vi "SetUpGage.vi"(0 "Digitizer Settings":T1={"Digitizer delay (us) "=0.0, "rf points per line"=2048, "lines per plane"=128, "Samp Rate (Hz)"=100000000.0, "Additional dig delay (us)"=0.0, "Voltage Scale"=0.4, "Pre-Looks"=0, "Offset delay (us)"=0.0, "bits A/D"=8, "Avg Num"=1, "DigTimeOut"=5.0, "Rel Dig Delay"=0.0, "Dig Ch"=0, "LeCroyCluster"={"LeCroy Channels"=[TRUE, FALSE, FALSE, FALSE], "LC read pt offset"=0.0, "Sweep Avg"=FALSE}, "Main Digitizer"=enum."NI Digitizer", "Dig Config"=enum."Single channel", "Digitizer ID Cluster"={"Acqiris/Alazar/SP ID"=[], "NI Instr Handles"=[], "LeCroy VISA"="", "GaGe Handle"={"Handle"=0, "Sample size"=0, "Resolution"=0, "Offset"=0, "Channels"=0, "Boards"=0}, "ATS Ref"="ATS9350", "Acqiris Address"=["PCI::INSTR0"], "ADQRef"=refnum, "adq_cu_ptr"=refnum}, "Trigger Settings"={"Trig Source"=1, "Trig Coupling"=0, "Trig Slope"=0, "Level (mV)"=1500.0}, "Bulk Acq"=FALSE, "Bulk Start Indexes"=[], "Data Ref RF"=refnum, "NI ID/Channel"=[], "Total Dig CH"=5, "Xtra Ann Trig delay (us)"=10.0, "Fix Z Delay?"=FALSE, "One Way Transmission?"=FALSE, "Data Ref Log"=refnum} {"Trigger Settings"."Trig Slope" items=["Positive", "Negative"]; "Trigger Settings"."Level (mV)" format="%.2f"; "Trigger Settings"."Trig Coupling" items=["DC 1 MOhm", "AC 1 MOhm", "DC 50 Ohm", "AC 50 Ohm"]; "Trigger Settings"."Trig Source" items=["Chan 1", "External"]; "Rel Dig Delay" format="%.2f"; "DigTimeOut" format="%.2f"; "Avg Num" min=1; "Offset delay (us)" format="%.2f"; "Additional dig delay (us)" format="%.2f"; "Digitizer delay (us)" format="%.2f"}, 1 "Vecchio Hitachi?":bool, 3 "Acquisition In":T5, 4 "Attenuation":u8(slide) max=63 scale=0.0..63.0, 5 "Vector Trigger Line":i16=150 min=2 max=315, 6 "Machine Type":enum16{"Hitachi", "B&K 3535", "B&K Hawk"}(ring)) -> (12 "Total Delay (ms)":dbl format="%.2f", 13 "Additional dig delay (ms) out":dbl format="%.2f", 14 "Digitizer Settings Out":T1={"Digitizer delay (us) "=0.0, "rf points per line"=2048, "lines per plane"=128, "Samp Rate (Hz)"=100000000.0, "Additional dig delay (us)"=0.0, "Voltage Scale"=0.4, "Pre-Looks"=0, "Offset delay (us)"=0.0, "bits A/D"=8, "Avg Num"=1, "DigTimeOut"=5.0, "Rel Dig Delay"=0.0, "Dig Ch"=0, "LeCroyCluster"={"LeCroy Channels"=[TRUE, FALSE, FALSE, FALSE], "LC read pt offset"=0.0, "Sweep Avg"=FALSE}, "Main Digitizer"=enum."NI Digitizer", "Dig Config"=enum."Single channel", "Digitizer ID Cluster"={"Acqiris/Alazar/SP ID"=[], "NI Instr Handles"=[], "LeCroy VISA"="", "GaGe Handle"={"Handle"=0, "Sample size"=0, "Resolution"=0, "Offset"=0, "Channels"=0, "Boards"=0}, "ATS Ref"="ATS9350", "Acqiris Address"=["PCI::INSTR0"], "ADQRef"=refnum, "adq_cu_ptr"=refnum}, "Trigger Settings"={"Trig Source"=1, "Trig Coupling"=0, "Trig Slope"=0, "Level (mV)"=1500.0}, "Bulk Acq"=FALSE, "Bulk Start Indexes"=[], "Data Ref RF"=refnum, "NI ID/Channel"=[], "Total Dig CH"=5, "Xtra Ann Trig delay (us)"=10.0, "Fix Z Delay?"=FALSE, "One Way Transmission?"=FALSE, "Data Ref Log"=refnum} {"Trigger Settings"."Trig Slope" items=["Positive", "Negative"]; "Trigger Settings"."Level (mV)" format="%.2f"; "Trigger Settings"."Trig Coupling" items=["DC 1 MOhm", "AC 1 MOhm", "DC 50 Ohm", "AC 50 Ohm"]; "Trigger Settings"."Trig Source" items=["Chan 1", "External"]; "Rel Dig Delay" format="%.2f"; "DigTimeOut" format="%.2f"; "Avg Num" min=1; "Offset delay (us)" format="%.2f"; "Additional dig delay (us)" format="%.2f"; "Digitizer delay (us)" format="%.2f"}, 15 "Attenuation out":u8, 16 "Acquisition Settings Out":T5, 18 "Equivalent round trip\ndelay distance (mm)":dbl format="%.2f", 19 "Voltage Scale (pp) OUT":i16(ring)=5)   [LabVIEW 2022 SP3]
uses:
  <vilib>/Analysis/NI_AALPro.lvlib
  <instrlib>/vi.lib/Platform/portaccess.llb/Out Port8.vi
  <vilib>/Analysis/NI_AALBase.lvlib
  <vilib>/Analysis/baseanly.llb/Mean (DBL).vi
  ProstateDataAcq/-ProstateScanSystem/RFSamplingCluster.ctl
  -DigitizerRoutines/DigitizerID.ctl
  -DigitizerRoutines/DigitizerSettings.ctl
  -DigitizerRoutines/Digitizer.ctl
  -DigitizerRoutines/DigConfig.ctl
  C:/Windows/System32/ADQAPI_dotNet_helper.dll
panel:
  in  "Trigger Settings":T6={"Source"=1, "Coupling"=0, "Slope"=0, "Level (mV)"=1500.0} {"Slope" items=["Positive", "Negative"]; "Level (mV)" format="%.2f"; "Coupling" items=["DC 1 MOhm", "AC 1 MOhm", "DC 50 Ohm", "AC 50 Ohm"]; "Source" items=["Chan 1", "External"]}
  in  "Offset (mV)":dbl
  in  "Channel":u16(ring) items=["Ch 0", "Ch 1"]
  in  "Voltage Scale (pp)":i16(ring)=5
  in  "go to scan type":bool
  in  "ExitSendCmd":bool
  in  "Coupling":u16(ring)=3 items=["DC 1 MOhm", "AC 1 MOhm", "DC 50 Ohm", "AC 50 OHM"]
  in  "Time scale per Div":i32(ring)=7 items=["100 ns", "200 ns", "500 ns", "1 micros", "2 micros", "5 micros", "10 micros", "20 micros", "50 micros", "100 micros", "200 micros"]
  out "Waveform\nGraph":cluster{i32, dbl, dbl[]}(graph)
  out "Error Message":string
  in  "RF data Sampling":T7={"Sampling Rate"=50, "Ref Delay (ms)"=0.0, "rf points per line"=2500} {"Ref Delay (ms)" format="%.2f"}
  # "Digitizer Settings"
  # "Scale Settings"
  # "Need to autoscale if viewing spectrum. Yellow curser used for additional delay.\nRF data is captured between yellow and red lines."
  # "© 2000-2014 Riverside Research Institute"
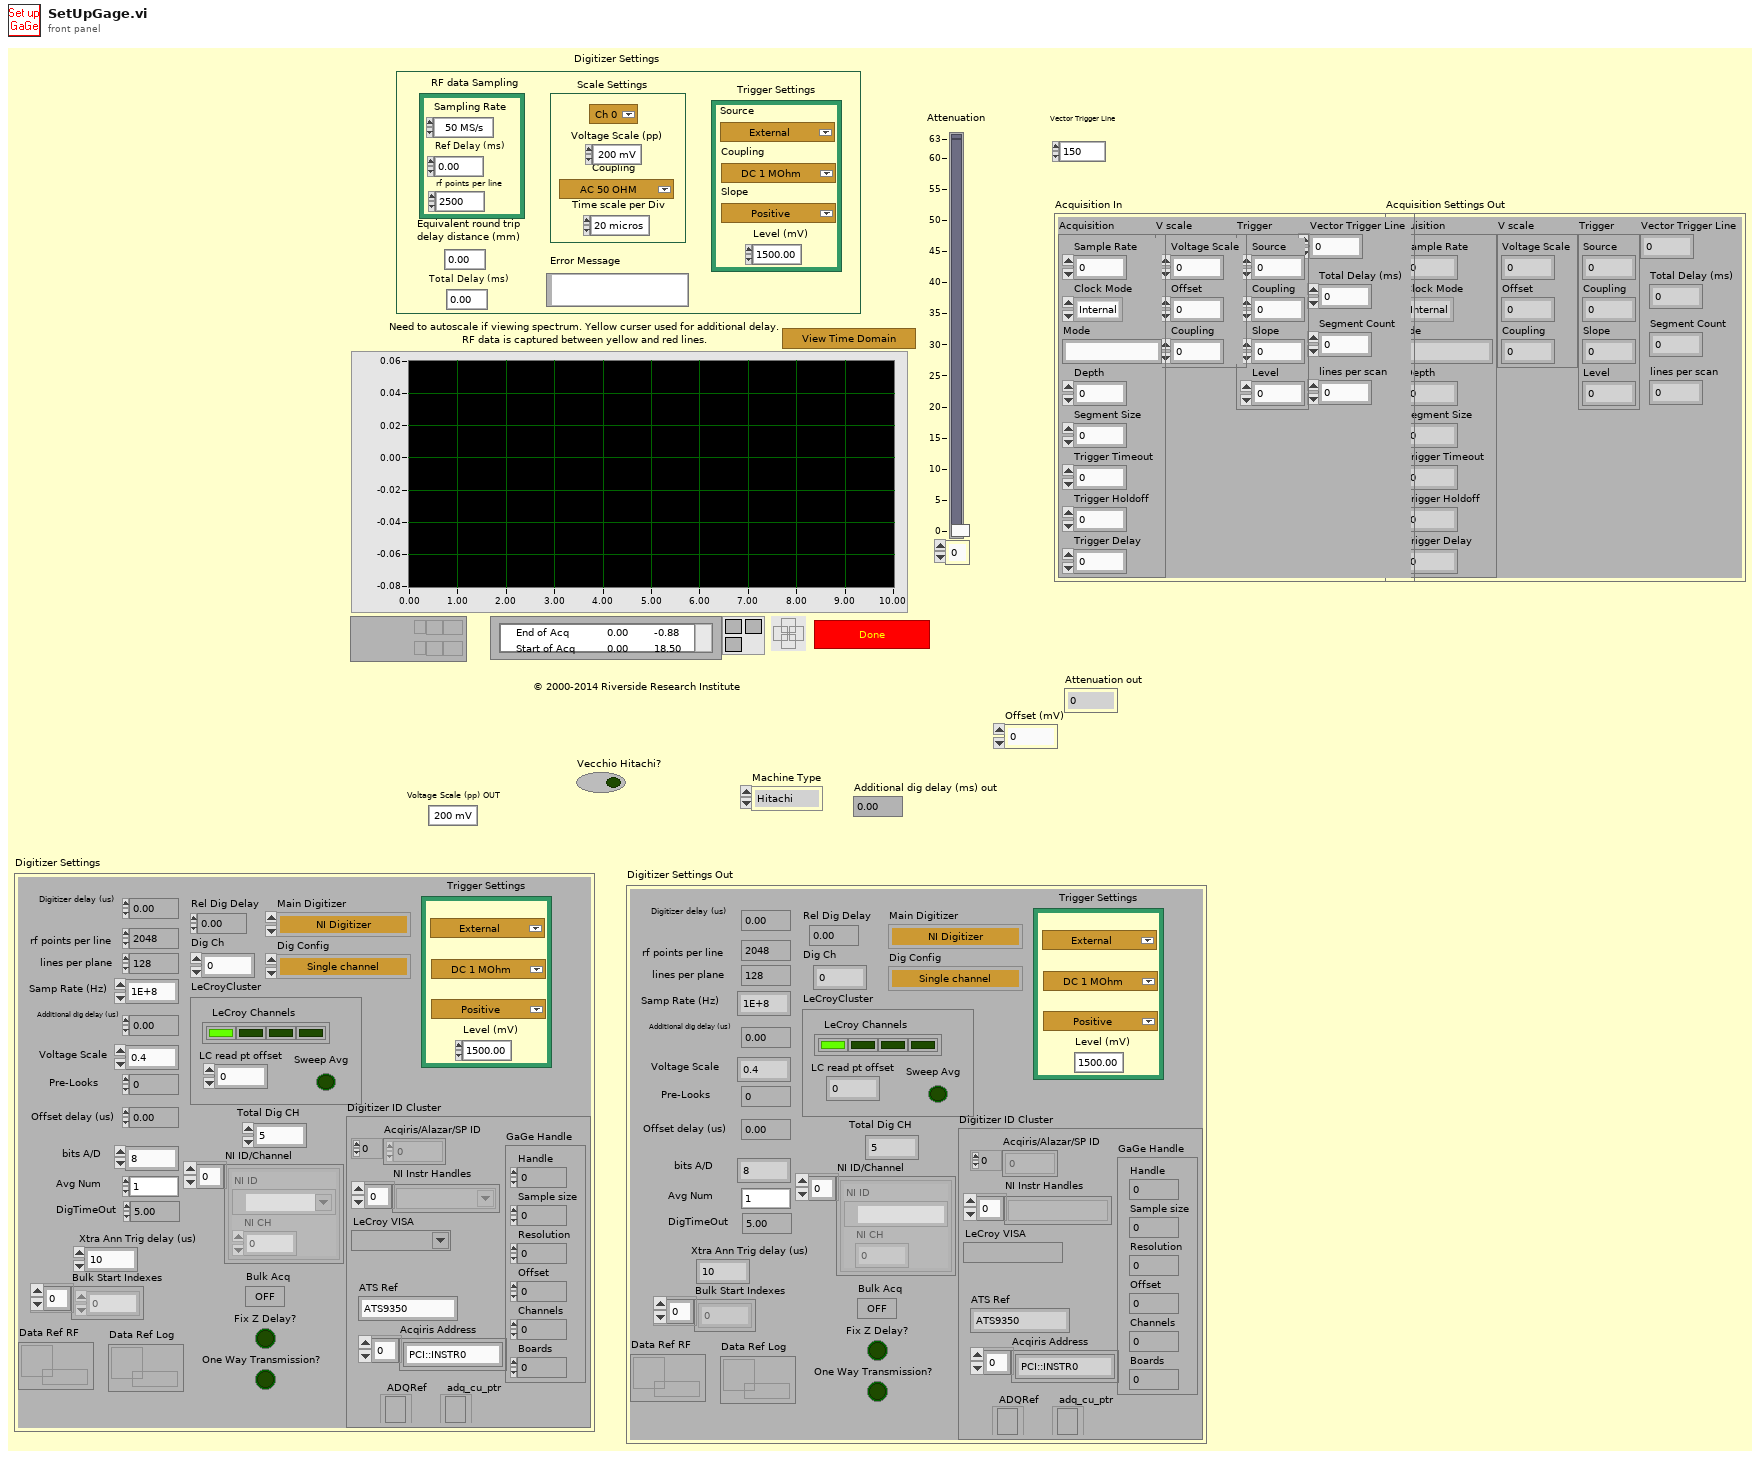
[diagram p1: front panel]
types:
  T1 = typedef "DigitizerSettings.ctl" = cluster{"Digitizer delay (us) ":dbl, "rf points per line":i32, "lines per plane":i32, "Samp Rate (Hz)":dbl, "Additional dig delay (us)":dbl, "Voltage Scale":dbl, "Pre-Looks":i32, "Offset delay (us)":dbl, "bits A/D":i8, "Avg Num":i32, "DigTimeOut":sgl, "Rel Dig Delay":sgl, "Dig Ch":i32, "LeCroyCluster":cluster{"LeCroy Channels":bool[], "LC read pt offset":dbl, "Sweep Avg":bool}, "Main Digitizer":T2, "Dig Config":T3, "Digitizer ID Cluster":T4, "Trigger Settings":cluster{"Trig Source":u16, "Trig Coupling":u16, "Trig Slope":u16, "Level (mV)":dbl}, "Bulk Acq":bool, "Bulk Start Indexes":i32[], "Data Ref RF":refnum<data-value>, "NI ID/Channel":cluster{"NI ID":refnum<k15>, "NI CH":i32}[], "Total Dig CH":i32, "Xtra Ann Trig delay (us)":dbl, "Fix Z Delay?":bool, "One Way Transmission?":bool, "Data Ref Log":refnum<data-value>}
  T2 = typedef "Digitizer.ctl" = enum16{"Acqiris Digitizer", "NI Digitizer", "LeCroy", "GaGe", "AlazarTech", "No Digitizer", "Teledyne"}
  T3 = typedef "DigConfig.ctl" = enum16{"Single channel", "2 Chans w/ 2 Acqiris", "2 Chans w/ 1 Acqiris", "5-CH Pulser New", "5-CH pulser w/ ann array", "5-pass style ann array", "Empty"}
  T4 = typedef "DigitizerID.ctl" = cluster{"Acqiris/Alazar/SP ID":u32[], "NI Instr Handles":refnum<k15>[], "LeCroy VISA":refnum<visa-resource-name>, "GaGe Handle":cluster{"Handle":u32, "Sample size":u32, "Resolution":i32, "Offset":i32, "Channels":u32, "Boards":u32}, "ATS Ref":string, "Acqiris Address":string[], "ADQRef":refnum<k24>, "adq_cu_ptr":refnum<k24>}
  T5 = cluster{"Acquisition":cluster{"Sample Rate":dbl, "Clock Mode":enum16{"Internal", "External", "Reference"}, "Mode":string, "Depth":dbl, "Segment Size":dbl, "Trigger Timeout":dbl, "Trigger Holdoff":dbl, "Trigger Delay":dbl}, "V scale":cluster{"Voltage Scale":i16, "Offset":dbl, "Coupling":u16}, "Trigger":cluster{"Source":u16, "Coupling":u16, "Slope":u16, "Level":dbl}, "Vector Trigger Line":i16, "Total Delay (ms)":dbl, "Segment Count":u32, "lines per scan":i32}
  T6 = cluster{"Source":u16, "Coupling":u16, "Slope":u16, "Level (mV)":dbl}
  T7 = typedef "RFSamplingCluster.ctl" = cluster{"Sampling Rate":u16, "Ref Delay (ms)":dbl, "rf points per line":u16}
  T8 = cluster{"Handle":u32, "Sample size":u32, "Resolution":i32, "Offset":i32, "Channels":u32, "Boards":u32}
  T9 = cluster{"Voltage Scale (pp)":i16, dbl, "Coupling":u16}
  T10 = cluster{"Sample Rate":dbl, "Clock Mode":enum16{"Internal", "External", "Reference"}, "Mode":string, "Depth":dbl, "Segment Size":dbl, "Trigger Timeout":dbl, "Trigger Holdoff":dbl, "Trigger Delay":dbl}
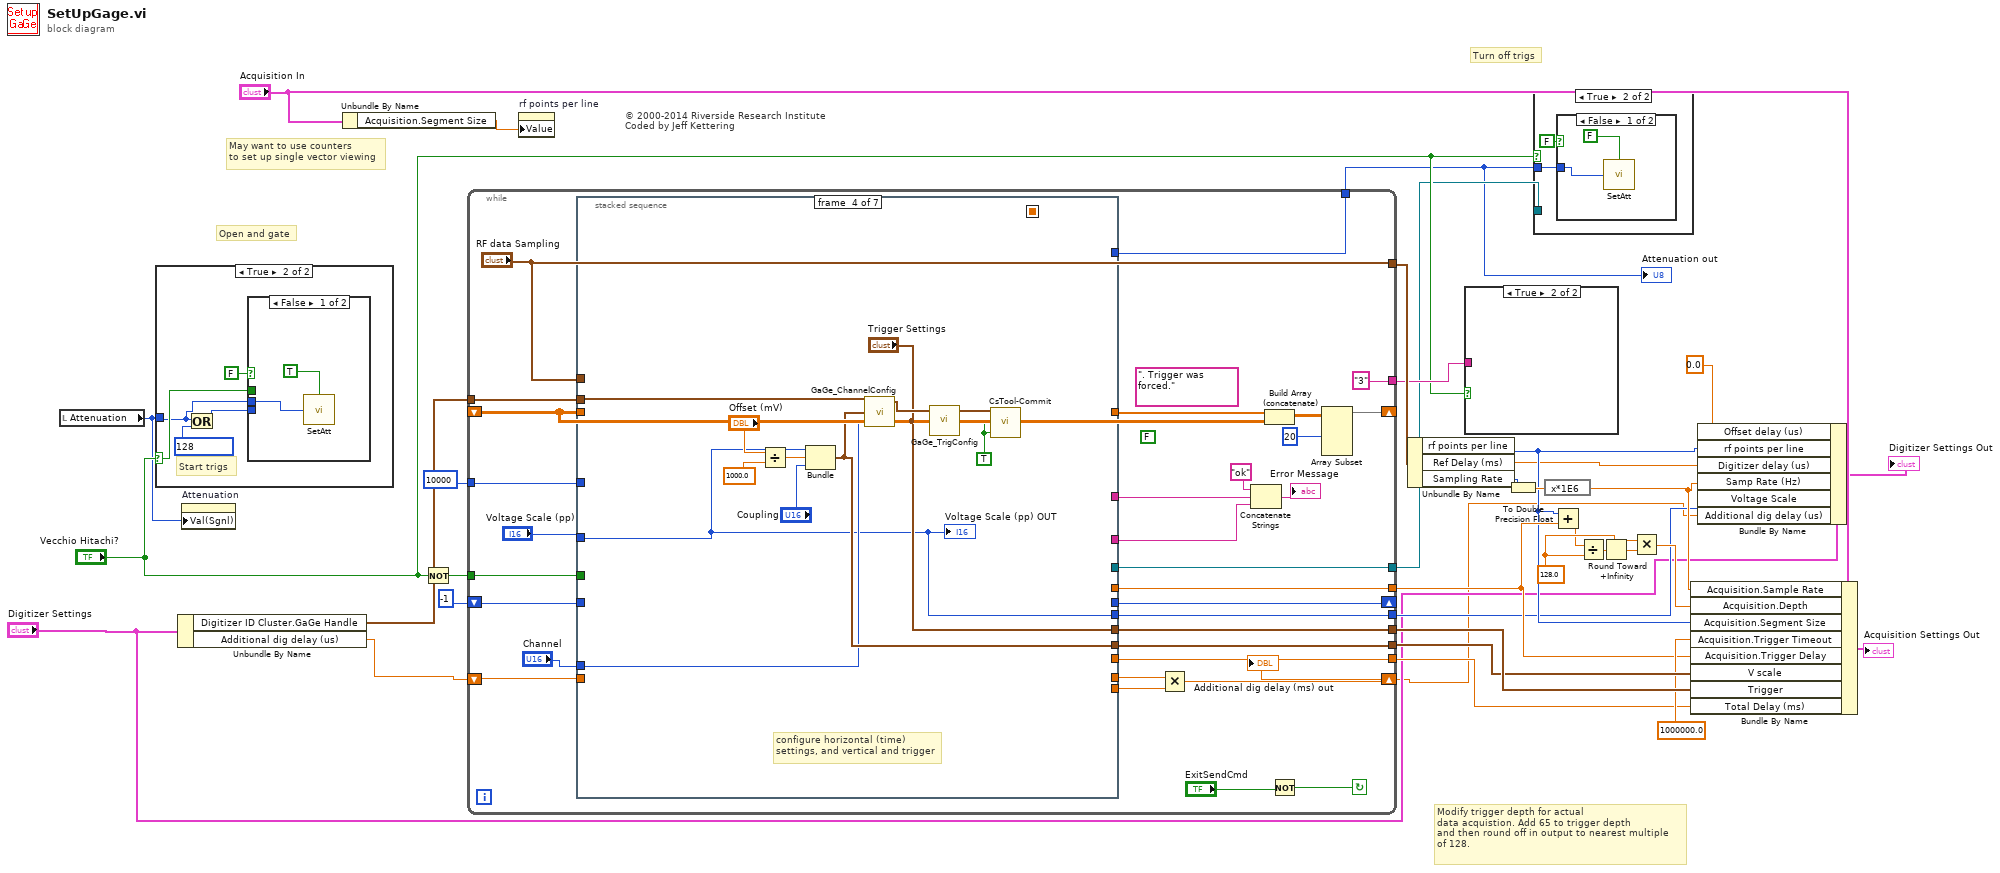
[diagram p0: block diagram]
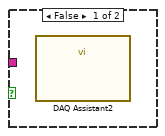
[diagram p2: hidden frame]
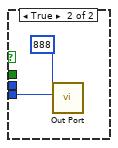
[diagram p4: hidden frame]
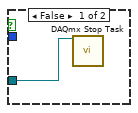
[diagram p5: hidden frame]
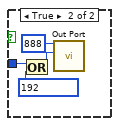
[diagram p6: hidden frame]
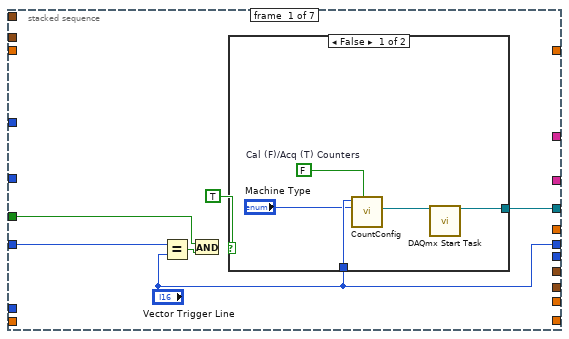
[diagram p7: hidden frame]
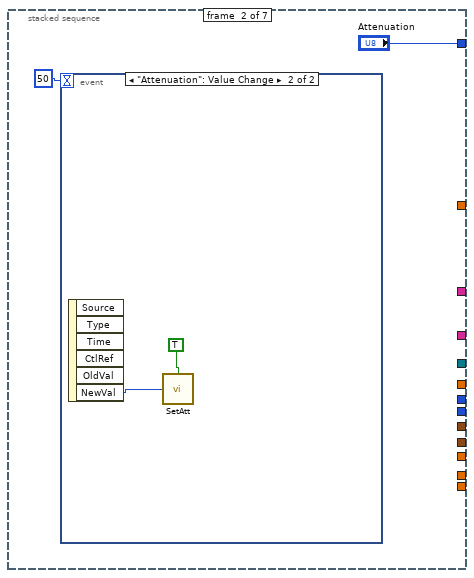
[diagram p9: hidden frame]
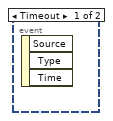
[diagram p10: hidden frame]
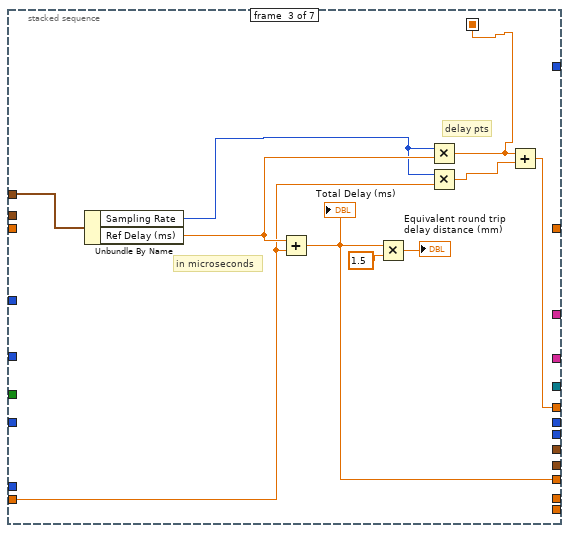
[diagram p11: hidden frame]
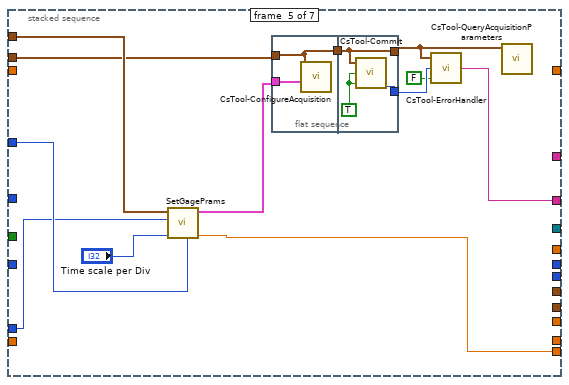
[diagram p12: hidden frame]
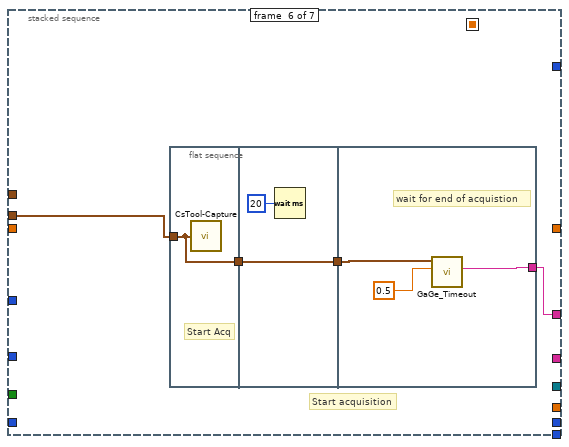
[diagram p13: hidden frame]
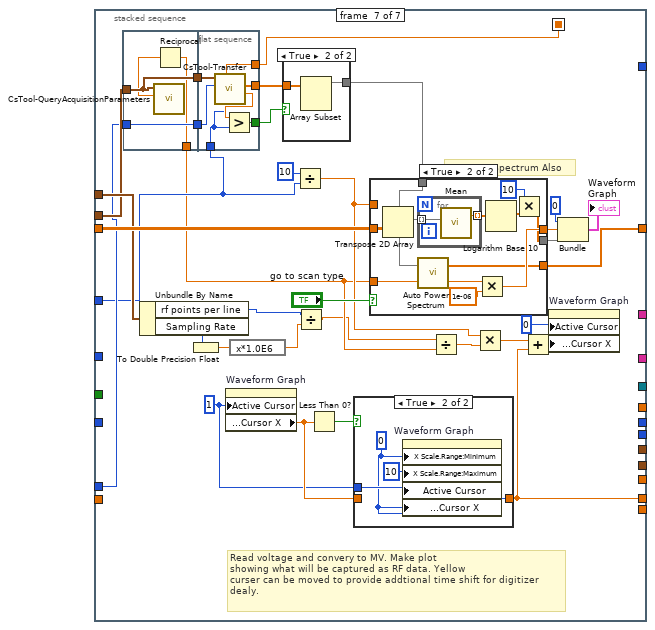
[diagram p14: hidden frame]
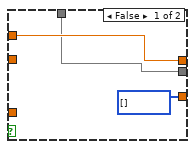
[diagram p17: hidden frame]
diagram:
  w18 = 128.0 ("y")
  # "© 2000-2014 Riverside Research Institute\nCoded by Jeff Kettering"
  # "Turn off trigs"
  # "Open and gate"
  # "May want to use counters\nto set up single vector viewing"
  # "Modify trigger depth for actual\ndata acquistion. Add 65 to trigger depth\nand then round off in output to nearest multiple\nof 128."
  n1 = local read "Attenuation"() -> (w11:u8)
  n2 = case shown="True" "Vecchio Hitachi?" {
    selector: "Vecchio Hitachi?" -> [_ w36]
    tunnel: w11 -> [_ w35]
    frame False {
    }
    frame True {
      # "Start trigs"
      n3 = Or(x=w35, y=u8 128) -> (x .or. y?=w38:u8)
      n4 = case shown="False" FALSE {
        tunnel: w38 -> [_ w42]
        tunnel: w36 -> [_ _]
        tunnel: w35 -> [w41 _]
        frame False {
          n5 = call "SetAtt.vi"("Arm Trigs?"=TRUE, "Attenuation"=w41) -> ()  [unwired: 4 in]
        }
        frame True {
          n6 = call-poly <instrlib>:"Out Port.vi"("write value"=w42, "address"=u32 888 ("Port Address")) -> ()  [unwired: 1 in, 7 out]
        }
      }
    }
  }
  n7 = Unbundle By Name("Digitizer Settings") -> ("Digitizer ID Cluster.GaGe Handle"=w10:T8, "Additional dig delay (us)"=w9:dbl)
  n8 = property on="Attenuation" class="Slide (strict)"("Val(Sgnl)"=w11) -> ()  [unwired: 2 in, 2 out]
  n9 = Unbundle By Name("Acquisition In") -> ("Acquisition.Segment Size"=w23:dbl)
  n10 = Not(x="Vecchio Hitachi?") -> (.not. x?=w32:bool)
  n11 = while {
    tunnel: [w57] -> w17
    shift-left: -1 -> [w59]
    shift-right: [w58] -> _
    shift-left: _ -> [w69]
    shift-right: [w67] -> _
    shift-left: w9 -> [w70]
    shift-right: [w63] -> w1
    tunnel: ["RF data Sampling"] -> w34
    tunnel: w32 -> [w56]
    tunnel: ["3" ("counter")] -> w31
    tunnel: [w54] -> w29
    tunnel: w10 -> [w53]
    tunnel: [w51] -> w28
    tunnel: [w50] -> w27
    tunnel: [w49] -> w15
    tunnel: 10000 -> [w48]
    tunnel: [w45] -> w13
    tunnel: [w44] -> w4
    stop <- w72 continue-if-true
    (unwired) FALSE
    (unwired) ". Trigger was forced."
    n12 = stacked-sequence {
      seq-local: [_ _ w91 _ _ _ _] -> [_ _ _ _ _ _ w144]
      tunnel: "RF data Sampling" -> [_ _ w97 _ w118 _ w158]
      tunnel: w70 -> [_ _ w95 _ _ _ _]
      tunnel: w69 -> [_ _ _ _ _ _ w161]
      tunnel: [_ _ _ _ _ _ w157] -> w60
      tunnel: [_ _ _ _ _ _ w159] -> w65
      tunnel: [_ _ _ _ w115 _ _] -> w64
      tunnel: "Voltage Scale (pp)" -> [_ _ _ w100 _ _ _]
      tunnel: w59 -> [w80 _ _ _ _ _ _]
      tunnel: ["Vector Trigger Line" _ _ _ _ _ _] -> w58
      tunnel: [_ _ w94 _ _ _ _] -> w57
      tunnel: "Channel" -> [_ _ _ w101 w112 _ w151]
      tunnel: w56 -> [w77 _ _ _ _ _ _]
      tunnel: [w76 _ _ _ _ _ _] -> w54
      tunnel: w53 -> [_ _ _ w108 w116 w130 w152]
      tunnel: [_ _ _ _ w120 _ _] -> w52
      tunnel: [_ _ _ "Trigger Settings" _ _ _] -> w51
      tunnel: [_ _ _ w102 _ _ _] -> w50
      tunnel: [_ _ w93 _ _ _ _] -> w49
      tunnel: w48 -> [_ _ _ _ w114 _ w146]
      tunnel: [_ _ _ _ _ w129 _] -> w47
      tunnel: [_ "Attenuation" _ _ _ _ _] -> w45
      tunnel: [_ _ _ w100 _ _ _] -> w44
      frame #0 {
        n13 = Equal?(x=w80, y="Vector Trigger Line") -> (x = y?=w78:bool)
        n14 = And(x=w77, y=w78) -> ()  [unwired: 1 out]
        n15 = case shown="False" TRUE {
          tunnel: "Vector Trigger Line" -> [w85 _]
          tunnel: [w81 _] -> w76
          frame False {
            w84 = FALSE  # Cal (F)/Acq (T) Counters
            n16 = call "CountConfig.vi"("Cal (F)/Acq (T) Counters"=w84, "Machine Type"="Machine Type", "pulse delay  (cycles)"=w85) -> ("task out"=w82:refnum<k21>)  [unwired: 8 out]
            n17 = call <vilib>:"DAQmx Start Task.vi"("task/channels in"=w82) -> ("task out"=w81:refnum<k21>)  [unwired: 1 in, 13 out]
          }
          frame True {
          }
        }
      }
      frame #1 {
        n18 = event shown="[1] \"Attenuation\": Value Change" {
          selector: _ -> [_ _]
          dyn-events: _ -> [_ _]
          timeout: 50 -> [_ _]
          event Timeout {
            n19 = event-data() -> ()  [unwired: 1 in, 3 out]
          }
          event "Attenuation": Value Change {
            n20 = event-data() -> ("NewVal"=w88:u8)  [unwired: 1 in, 5 out]
            n21 = call "SetAtt.vi"("Arm Trigs?"=TRUE ("Vecchio Hitachi?"), "Attenuation"=w88) -> ()  [unwired: 1 in, 3 out]
          }
        }
      }
      frame #2 {
        # "delay pts"
        # "in microseconds"
        n22 = Unbundle By Name(w97) -> ("Sampling Rate"=w90:u16, "Ref Delay (ms)"=w96:dbl)
        n23 = Add(x=w96, y=w95) -> (x+y=w94:dbl)
        "Total Delay (ms)" <- w94
        n24 = Multiply(x=w94, y=1.5) -> (x*y=→"Equivalent round trip\ndelay distance (mm)":dbl)
        n25 = Multiply(x=w90, y=w96) -> (x*y=w91:dbl)
        n26 = Multiply(x=w90, y=w95) -> (x*y=w92:dbl)
        n27 = Add(x=w91, y=w92) -> (x+y=w93:dbl)
      }
      frame #3 {
        w110 = TRUE
        # "configure horizontal (time)\nsettings, and vertical and trigger"
        n28 = Divide(x="Offset (mV)", y=1000.0 ("x")) -> (x/y=w105:dbl)
        n29 = Bundle("Voltage Scale (pp)"=w100, w105, "Coupling"="Coupling") -> (w102:T9)  [unwired: 1 out]
        n30 = call "GaGe_ChannelConfig.vi"("Channel (0)"=w101, "V scale"=w102, "Handle Cluster"=w108) -> ("Handle Cluster Out"=w111:T8)  [unwired: 2 in]
        n31 = call "GaGe_TrigConfig.vi"("Trigger"="Trigger Settings", "Handle Cluster"=w111) -> ("Handle Cluster Out"=w109:T8)  [unwired: 3 in]
        n32 = call <userlib>:"CsTool-Commit.vi"("OnlyOnChange (t)"=w110, "Coerce Flag (f)"=w110, "Handle Cluster"=w109) -> ()  [unwired: 2 out]
        "Voltage Scale (pp) OUT" <- w100
      }
      frame #4 {
        n33 = call "SetGagePrams.vi"("Pts to take"=w114, "Time scale per Div"="Time scale per Div", "Channel"=w112, "RF data Sampling"=w118) -> ("Time per division"=w115:dbl, "Temp Set Up Digi Params"=w113:T10)  [unwired: 5 in, 1 out]
        n34 = flat-sequence {
          tunnel: w113 -> [w125]
          tunnel: w116 -> [w124]
          tunnel: [w124] -> w123
          tunnel: w123 -> [w127]
          tunnel: [w127] -> w117
          tunnel: [w126] -> w122
          frame #0 {
            n35 = call <userlib>:"CsTool-ConfigureAcquisition.vi"("Handle Cluster"=w124, "Acquisition"=w125) -> ()  [unwired: 3 in, 1 out]
          }
          frame #1 {
            w128 = TRUE
            n36 = call <userlib>:"CsTool-Commit.vi"("OnlyOnChange (t)"=w128, "Coerce Flag (f)"=w128, "Handle Cluster"=w127) -> ("Error Code"=w126:i32)  [unwired: 1 out]
          }
        }
        n37 = call <userlib>:"CsTool-ErrorHandler.vi"("StopOnError (true)"=FALSE, "Error Code"=w122, "Handle Cluster"=w117) -> ("Error String"=w120:string)
        n38 = call <userlib>:"CsTool-QueryAcquisitionParameters.vi"("Handle Cluster"=w117) -> ()  [unwired: 11 out]
      }
      frame #5 {
        # "Start acquisition"
        n39 = flat-sequence {
          tunnel: w130 -> [w133]
          tunnel: [w133] -> w132
          tunnel: w132 -> [w135]
          tunnel: [w135] -> w131
          tunnel: w131 -> [w138]
          tunnel: [w137] -> w129
          frame #0 {
            # "Start Acq"
            n40 = call <userlib>:"CsTool-Capture.vi"("Handle Cluster"=w133) -> ()  [unwired: 1 out]
          }
          frame #1 {
            n41 = Wait (ms)(milliseconds to wait=u32 20) -> ()  [unwired: 1 out]
          }
          frame #2 {
            # "wait for end of acquistion"
            n42 = call "GaGe_Timeout.vi"("TimeOut (s)"=sgl 0.5, "GaGe Handle"=w138) -> ("String"=w137:string)  [unwired: 8 in, 1 out]
          }
        }
      }
      frame #6 {
        w162 = u32 1 ("Write Attribute")
        # "Can View Spectrum Also"
        # "Read voltage and convery to MV. Make plot\nshowing what will be captured as RF data. Yellow\ncurser can be moved to provide addtional time shift for digitizer\ndealy."
        n43 = flat-sequence {
          tunnel: w152 -> [w178]
          tunnel: w151 -> [w176]
          tunnel: [w178] -> w156
          tunnel: [w176] -> w155
          tunnel: [w175] -> w145
          tunnel: [w185] -> w154
          tunnel: w156 -> [w184]
          tunnel: w146 -> [w181]
          tunnel: w155 -> [w179]
          tunnel: [w183] -> w153
          tunnel: w144 -> [w180]
          frame #0 {
            n44 = call <userlib>:"CsTool-QueryAcquisitionParameters.vi"("Handle Cluster"=w178) -> ("Sample Rate"=w177:dbl)  [unwired: 10 out]
            n45 = Reciprocal(x=w177) -> (1/x=w175:dbl)
          }
          frame #1 {
            n46 = call <userlib>:"CsTool-Transfer.vi"("Length (4096)"=w181, "Start (0)"=w180, "Channel (0)"=w179, "Handle Cluster"=w184) -> ("Actual Length"=w182:dbl, "Data in Volts"=w185:dbl[])  [unwired: 2 in, 2 out]
            n47 = Greater?(x=w182, y=w181) -> (0:w183:bool)
          }
        }
        n48 = Unbundle By Name(w158) -> ("rf points per line"=w143:u16, "Sampling Rate"=w142:u16)
        n49 = To Double Precision Float(number=w142) -> (double precision float=w139:dbl)
        n50 = property on="Waveform Graph" class="WFGraph (strict)"("Active Cursor"=w162) -> ("Cursor.Cursor Position:Cursor X"=w165:dbl)  [unwired: 2 in, 2 out]
        n51 = expression code="x*1.0E6"(w139) -> (w141:dbl)
        n52 = case shown="True" w153 {
          tunnel: [w172 w174] -> w150
          tunnel: w154 -> [w172 w173]
          frame False {
          }
          frame True {
            n53 = Array Subset(array=w173) -> (w174:dbl[])  [unwired: 2 in]
          }
        }
        n54 = Divide(x=10, y=w146) -> (x/y=w148:dbl)
        n55 = Divide(x=w143, y=w141) -> (x/y=w140:dbl)
        n56 = Less Than 0?(x=w165) -> (x < 0?=w163:bool)
        n57 = case shown="True" w163 {
          tunnel: w165 -> [w186 _]
          tunnel: [w186 w187] -> w159
          tunnel: w162 -> [_ w188]
          frame False {
          }
          frame True {
            w187 = 0
            n58 = property on="Waveform Graph" class="WFGraph (strict)"("X Scale.Range:Minimum"=w187, "X Scale.Range:Maximum"=10, "Active Cursor"=w188, "Cursor.Cursor Position:Cursor X"=w187) -> ()  [unwired: 2 in, 2 out]
          }
        }
        n59 = case shown="True" "go to scan type" {
          tunnel: [w190 w195] -> w160
          tunnel: w150 -> [w190 w194]
          tunnel: [w192 w201] -> w167
          tunnel: w148 -> [w192 _]
          tunnel: w145 -> [_ w204]
          tunnel: w161 -> [_ w200]
          tunnel: [i32[] [] w193] -> w157
          frame False {
          }
          frame True {
            n60 = Transpose 2D Array(2D array=w200) -> (transposed array=w199:dbl[][])
            n61 = for {
              tunnel: w199 -> [w206] mode=indexing
              tunnel: [w205] -> w198 mode=indexing
              n62 = call-poly <vilib>:"Mean.vi"("X"=w206) -> ("mean"=w205:dbl)  [unwired: 1 out]
            }
            n63 = call <vilib>:"Auto Power Spectrum.vi"("dt"=w204, "Signal (V)"=w194) -> ("df"=w203:dbl, "Power Spectrum (V^2 rms)"=w193:dbl[])
            n64 = Multiply(x=w203, y=1e-06) -> (x*y=w201:dbl)
            n65 = Logarithm Base 10(1:w198) -> (0:w196:dbl[])
            n66 = Multiply(x=10, y=w196) -> (x*y=w195:dbl[])
          }
        }
        n67 = Divide(x=w140, y=w145) -> (x/y=w149:dbl)
        n68 = Multiply(x=w148, y=w149) -> (x*y=w147:dbl)
        n69 = Add(x=w147, y=w159) -> (x+y=w164:dbl)
        n70 = property on="Waveform Graph" class="WFGraph (strict)"("Active Cursor"=0, "Cursor.Cursor Position:Cursor X"=w164) -> ()  [unwired: 2 in, 2 out]
        n71 = Bundle(0, w167, "Data in Volts"=w160) -> (→"Waveform\nGraph":cluster{i32, dbl, "Data in Volts":dbl[]})  [unwired: 1 out]
      }
    }
    n72 = Multiply(x=w65, y=w64) -> (x*y=w63:dbl)
    n73 = Concatenate Strings("ok", w47, w52) -> (→"Error Message":string)
    n74 = Build Array (concatenate)(w60, w69) -> (w68:dbl[][])
    n75 = Not(x="ExitSendCmd") -> (.not. x?=w72:bool)
    n76 = Array Subset(array=w68, length (row)=20) -> (w67:dbl[][])  [unwired: 3 in]
  }
  "Additional dig delay (ms) out" <- w1
  "Attenuation out" <- w13
  n77 = property on="rf points per line" class="DigNum (strict)"("Value"=w23) -> ()  [unwired: 2 in, 2 out]
  n78 = Unbundle By Name(w34) -> ("rf points per line"=w7:u16, "Ref Delay (ms)"=w6:dbl, "Sampling Rate"=w14:u16)
  n79 = case shown="True" "Vecchio Hitachi?" {
    tunnel: w31 -> [_ _]
    frame False {
      n80 = call "DAQ Assistant2"() -> ()  [unwired: 3 in, 17 out]
    }
    frame True {
    }
  }
  n81 = To Double Precision Float(number=w14) -> (double precision float=w12:dbl)
  n82 = case shown="True" "Vecchio Hitachi?" {
    tunnel: w13 -> [_ w209]
    tunnel: w29 -> [w207 _]
    frame False {
      n83 = call <vilib>:"DAQmx Stop Task.vi"("task/channels in"=w207) -> ()  [unwired: 1 in, 14 out]
    }
    frame True {
      n84 = case shown="False" FALSE {
        tunnel: w209 -> [w210 w213]
        frame False {
          n85 = call "SetAtt.vi"("Arm Trigs?"=FALSE ("Vecchio Hitachi?"), "Attenuation"=w210) -> ()  [unwired: 4 in]
        }
        frame True {
          n86 = Or(x=w213, y=u8 192) -> (x .or. y?=w212:u8)
          n87 = call-poly <instrlib>:"Out Port.vi"("write value"=w212, "address"=u32 888 ("Port Address")) -> ()  [unwired: 1 in, 7 out]
        }
      }
    }
  }
  n88 = expression code="x*1E6"(w12) -> (w5:dbl)
  n89 = Add(x=w7, y=w15) -> (x+y=w16:dbl)
  n90 = Divide(x=w16, y=w18) -> (x/y=w21:dbl)
  n91 = Round Toward +Infinity(x=w21) -> (ceil(x): smallest int >= x=w20:dbl)
  n92 = Multiply(x=w18, y=w20) -> (x*y=w19:dbl)
  n93 = Bundle By Name(cluster="Acquisition In", "Acquisition.Sample Rate"=w5, "Acquisition.Depth"=w19, "Acquisition.Segment Size"=w7, "Acquisition.Trigger Timeout"=1000000.0, "Acquisition.Trigger Delay"=w15, "V scale"=w27, "Trigger"=w28, "Total Delay (ms)"=w17) -> (→"Acquisition Settings Out":T5)
  n94 = Bundle By Name(cluster="Digitizer Settings", "Offset delay (us)"=0.0 ("Offset delay (ms)"), "rf points per line"=w7, "Digitizer delay (us)"=w6, "Samp Rate (Hz)"=w5, "Voltage Scale"=w4, "Additional dig delay (us)"=w1) -> (→"Digitizer Settings Out":T1)
